vi "orderbook.test.Modify.Order.3rd.of.3.vi"(8 "error in":errorcluster) -> (0 "error out":errorcluster, 3 "Passed":bool)   [LabVIEW 2022 SP3]
uses:
  arty/orderbook/orderbook.command.type.ctl
  arty/orderbook/orderbook.command.ctl
  fpga/app/orderbook.result.type.ctl
  fpga/app/orderbook.entry.ctl
panel:
  out "Counters":T1
  out "OrderBook.Entries":T2[](array[typedef]) {"Side (U8)" format="%.0x"}
  in  "OrderBook.Command[]\nto Send":T4[](array[typedef])=[{"OrderBook Command.Type"=enum."AddOrder", "Side (U8)"=66, "Order Id (U64)"=5290, "Quantity (U32)"=130, "Symbol (U64)"=29033, "Price (U64)"=9525, "Executed Quantity (U32)"=0, "Cancelled Quantity (U32)"=0}, {"OrderBook Command.Type"=enum."AddOrder", "Side (U8)"=66, "Order Id (U64)"=5291, "Quantity (U32)"=225, "Symbol (U64)"=29033, "Price (U64)"=9115, "Executed Quantity (U32)"=0, "Cancelled Quantity (U32)"=0}, {"OrderBook Command.Type"=enum."AddOrder", "Side (U8)"=0, "Order Id (U64)"=5292, "Quantity (U32)"=75, "Symbol (U64)"=29033, "Price (U64)"=9800, "Executed Quantity (U32)"=0, "Cancelled Quantity (U32)"=0}, {"OrderBook Command.Type"=enum."ModifyOrder", "Side (U8)"=66, "Order Id (U64)"=5290, "Quantity (U32)"=150, "Symbol (U64)"=0, "Price (U64)"=9525, "Executed Quantity (U32)"=0, "Cancelled Quantity (U32)"=0}, {"OrderBook Command.Type"=enum."Get.All.Orders", "Side (U8)"=0, "Order Id (U64)"=0, "Quantity (U32)"=0, "Symbol (U64)"=0, "Price (U64)"=0, "Executed Quantity (U32)"=0, "Cancelled Quantity (U32)"=0}] {"Side (U8)" format="%.0x"; "Order Id (U64)" format="%.0x"; "Symbol (U64)" format="%.0x"}
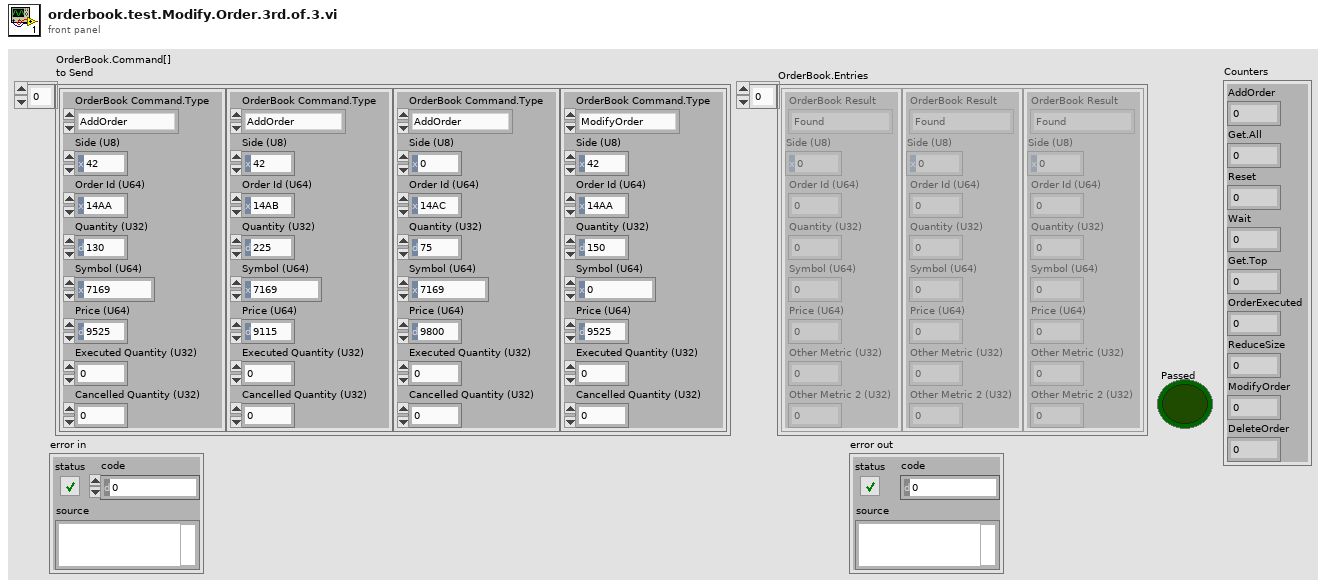
[diagram p1: front panel]
types:
  T1 = cluster{"AddOrder":u32, "Get.All":u32, "Reset":u32, "Wait":u32, "Get.Top":u32, "OrderExecuted":u32, "ReduceSize":u32, "ModifyOrder":u32, "DeleteOrder":u32}
  T2 = typedef "orderbook.entry.ctl" = cluster{"OrderBook Result":T3, "Side (U8)":u8, "Order Id (U64)":u64, "Quantity (U32)":u32, "Symbol (U64)":u64, "Price (U64)":u64, "Other Metric (U32)":u32, "Other Metric 2 (U32)":u32}
  T3 = typedef "orderbook.result.type.ctl" = enum16{"Found", "Not.Found"}
  T4 = typedef "orderbook.command.ctl" = cluster{"OrderBook Command.Type":T5, "Side (U8)":u8, "Order Id (U64)":u64, "Quantity (U32)":u32, "Symbol (U64)":u64, "Price (U64)":u64, "Executed Quantity (U32)":u32, "Cancelled Quantity (U32)":u32}
  T5 = typedef "orderbook.command.type.ctl" = enum16{"AddOrder", "OrderExecuted", "ReduceSize", "ModifyOrder", "DeleteOrder", "Get.All.Orders", "Get.Top"}
  T6 = cluster{"Write.Request":bool, "Read.Request":bool, "Read.Address":u32, "Read.OrderBook.Entry":cluster{"OrderBook Result":enum16{"Found", "Not.Found"}, "Side (U8)":u8, "Order Id (U64)":u64, "Quantity (U32)":u32, "Symbol (U64)":u64, "Price (U64)":u64, "Other Metric (U32)":u32, "Other Metric 2 (U32)":u32}, "Number.of.Entries":u32, "OrderBook.State":enum16{"Reset", "Wait", "Get.Top", "Get.All.Orders", "AddOrder", "Order.Executed", "Reduce.Size", "Modify.Order", "Delete.Order"}, "Ready.For.OrderBook.Command":bool, "Memory.State":enum16{"New", "Request.Data", "Append", "Data.Ready"}, "Move":bool, "Read.Valid":bool, "Write.Address":u32, "Write.OrderBook.Entry":cluster{"OrderBook Result":enum16{"Found", "Not.Found"}, "Side (U8)":u8, "Order Id (U64)":u64, "Quantity (U32)":u32, "Symbol (U64)":u64, "Price (U64)":u64, "Other Metric (U32)":u32, "Other Metric 2 (U32)":u32}, "OrderBook.Result.Valid":bool, "Append":bool, "Counters":cluster{"AddOrder":u32, "Get.All":u32, "Reset":u32, "Wait":u32, "Get.Top":u32, "OrderExecuted":u32, "ReduceSize":u32, "ModifyOrder":u32, "DeleteOrder":u32}}
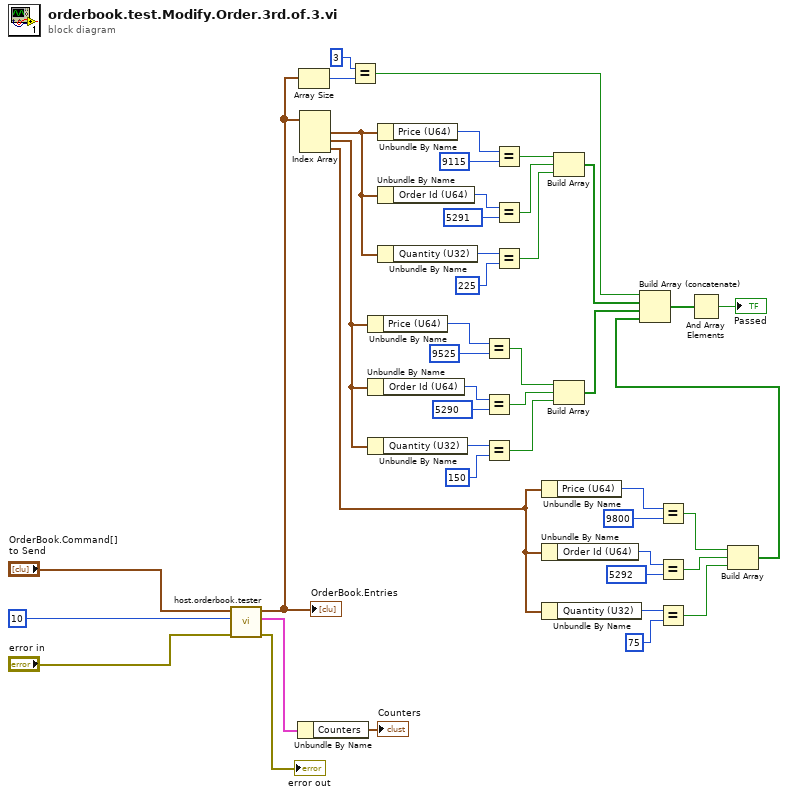
[diagram p0: block diagram]
diagram:
  n1 = call "host.orderbook.tester.vi"("error in"="error in", "Seconds to Wait"=10 ("Seconds\nto\nWait"), "OrderBook.Command[]\nto Send"="OrderBook.Command[]\nto Send") -> ("error out"=→"error out":errorcluster, "OrderBook.Variables"=w26:T6, "OrderBook.Entries"=w36:T2[])  [unwired: 6 in]
  "OrderBook.Entries" <- w36
  n2 = Unbundle By Name(w26) -> ("Counters"=→"Counters":T1)
  n3 = Array Size(array=w36) -> (size(s)=w42:i32)
  n4 = Index Array(array=w36) -> (element #1=w31:T2, element #2=w19:T2, element #3=w3:T2)  [unwired: 3 in]
  n5 = Equal?(x=3, y=w42) -> (x = y?=w13:bool)
  n6 = Unbundle By Name(w19) -> ("Price (U64)"=w25:u64)
  n7 = Unbundle By Name(w19) -> ("Order Id (U64)"=w23:u64)
  n8 = Unbundle By Name(w19) -> ("Quantity (U32)"=w21:u32)
  n9 = Unbundle By Name(w31) -> ("Price (U64)"=w39:u64)
  n10 = Unbundle By Name(w31) -> ("Order Id (U64)"=w34:u64)
  n11 = Unbundle By Name(w31) -> ("Quantity (U32)"=w30:u32)
  n12 = Equal?(x=w25, y=u64 9525) -> (x = y?=w16:bool)
  n13 = Equal?(x=w23, y=u64 5290) -> (x = y?=w17:bool)
  n14 = Equal?(x=w21, y=u32 150) -> (x = y?=w18:bool)
  n15 = Equal?(x=w39, y=u64 9115) -> (x = y?=w38:bool)
  n16 = Equal?(x=w34, y=u64 5291) -> (x = y?=w32:bool)
  n17 = Equal?(x=w30, y=u32 225) -> (x = y?=w28:bool)
  n18 = Unbundle By Name(w3) -> ("Price (U64)"=w12:u64)
  n19 = Unbundle By Name(w3) -> ("Order Id (U64)"=w10:u64)
  n20 = Unbundle By Name(w3) -> ("Quantity (U32)"=w8:u32)
  n21 = Build Array(w38, w32, w28) -> (w15:bool[])
  n22 = Build Array(w16, w17, w18) -> (w14:bool[])
  n23 = Equal?(x=w12, y=u64 9800) -> (x = y?=w4:bool)
  n24 = Equal?(x=w10, y=u64 5292) -> (x = y?=w5:bool)
  n25 = Equal?(x=w8, y=u32 75) -> (x = y?=w6:bool)
  n26 = Build Array(w4, w5, w6) -> (w2:bool[])
  n27 = Build Array (concatenate)(w13, w15, w14, w2) -> (w1:bool[])
  n28 = And Array Elements(Boolean array=w1) -> (logical AND=→"Passed":bool)
